vi "Template Retrieve Record.vi"(8 "error in (no error)":errorcluster, 11 "Statement Refnum":T1) -> (0 "error out":errorcluster, 2 "Template Record":T2, 3 "Statement Refnum":T1)   [LabVIEW 2011]
uses:
  Template Record.ctl
  Summitek EXT/ODBC/SQL Controls/Statement Refnum.ctl
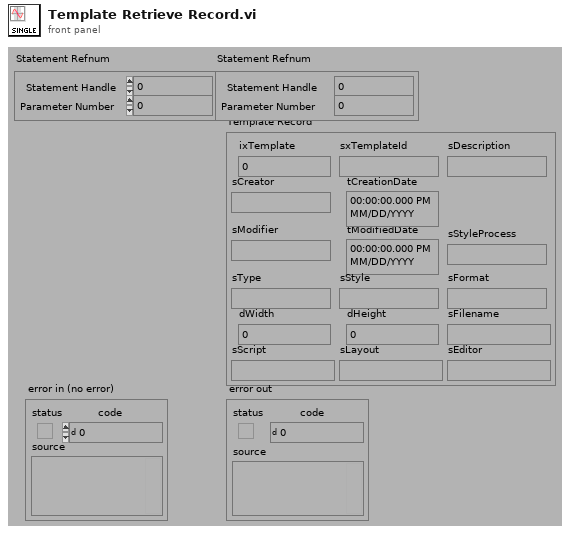
[diagram p1: front panel]
types:
  T1 = typedef "Statement Refnum.ctl" = cluster{"Statement Handle":i32, "Parameter Number":u16}
  T2 = typedef "Template Record.ctl" = cluster{"ixTemplate":i32, "sxTemplateId":string, "sDescription":string, "sCreator":string, "tCreationDate":timestamp, "sModifier":string, "tModifiedDate":timestamp, "sType":string, "sStyle":string, "sFormat":string, "dWidth":dbl, "dHeight":dbl, "sFilename":string, "sScript":string, "sLayout":string, "sEditor":string, "sStyleProcess":string}
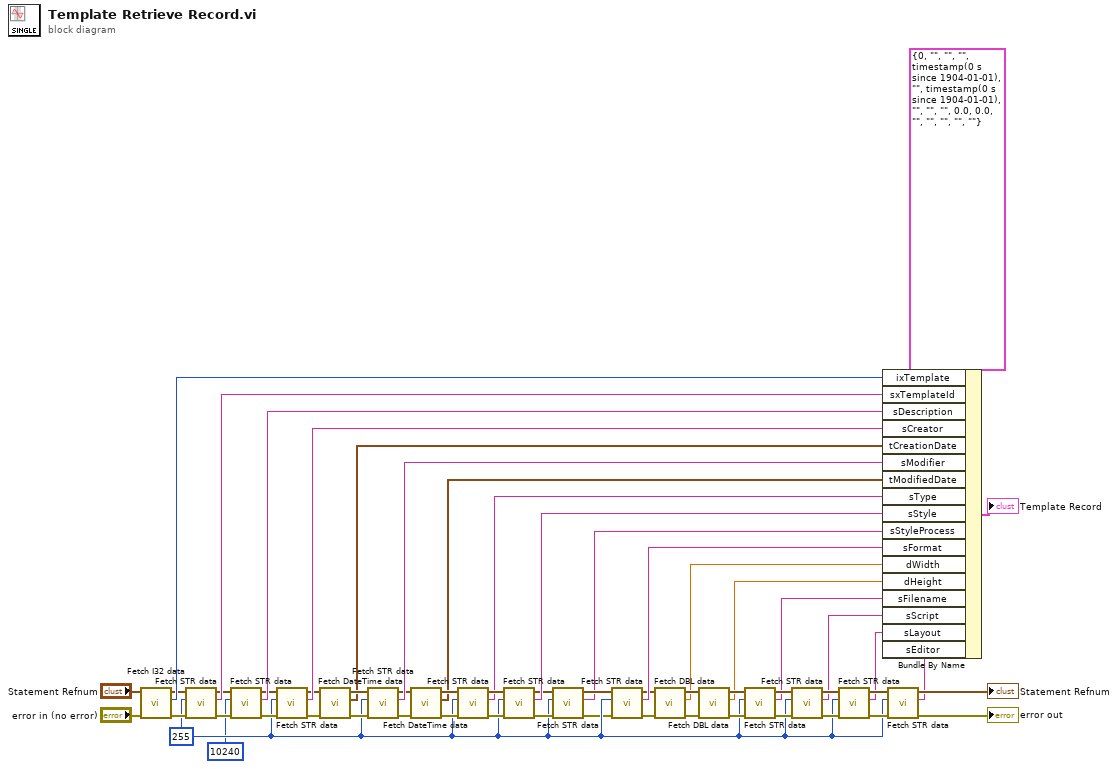
[diagram p0: block diagram]
diagram:
  w5 = 255 ("Buffer Size")
  n1 = call "Fetch I32 data.vi"("error in (no error)"="error in (no error)", "Statement Refnum"="Statement Refnum") -> ("error out"=w35:errorcluster, "Data"=w37:i32, "Statement Refnum"=w36:T1)  [unwired: 3 out]
  n2 = call "Fetch STR data.vi"("error in (no error)"=w35, "Buffer Size"=w5, "Statement Refnum"=w36) -> ("error out"=w33:errorcluster, "Data"=w34:string, "Statement Refnum"=w32:T1)  [unwired: 2 out]
  n3 = call "Fetch STR data.vi"("error in (no error)"=w33, "Buffer Size"=10240, "Statement Refnum"=w32) -> ("error out"=w30:errorcluster, "Data"=w31:string, "Statement Refnum"=w29:T1)  [unwired: 2 out]
  n4 = call "Fetch STR data.vi"("error in (no error)"=w30, "Buffer Size"=w5, "Statement Refnum"=w29) -> ("error out"=w26:errorcluster, "Data"=w28:string, "Statement Refnum"=w27:T1)  [unwired: 2 out]
  n5 = call "Fetch DateTime data.vi"("error in (no error)"=w26, "Statement Refnum"=w27) -> ("error out"=w51:errorcluster, "Data"=w25:timestamp, "Statement Refnum"=w50:T1)  [unwired: 3 out]
  n6 = call "Fetch STR data.vi"("error in (no error)"=w51, "Buffer Size"=w5, "Statement Refnum"=w50) -> ("error out"=w23:errorcluster, "Data"=w24:string, "Statement Refnum"=w22:T1)  [unwired: 2 out]
  n7 = call "Fetch DateTime data.vi"("error in (no error)"=w23, "Statement Refnum"=w22) -> ("error out"=w20:errorcluster, "Data"=w19:timestamp, "Statement Refnum"=w21:T1)  [unwired: 3 out]
  n8 = call "Fetch STR data.vi"("error in (no error)"=w20, "Buffer Size"=w5, "Statement Refnum"=w21) -> ("error out"=w54:errorcluster, "Data"=w16:string, "Statement Refnum"=w53:T1)  [unwired: 2 out]
  n9 = call "Fetch STR data.vi"("error in (no error)"=w54, "Buffer Size"=w5, "Statement Refnum"=w53) -> ("error out"=w6:errorcluster, "Data"=w18:string, "Statement Refnum"=w7:T1)  [unwired: 2 out]
  n10 = call "Fetch STR data.vi"("error in (no error)"=w6, "Buffer Size"=w5, "Statement Refnum"=w7) -> ("error out"=w3:errorcluster, "Data"=w2:string, "Statement Refnum"=w4:T1)  [unwired: 2 out]
  n11 = call "Fetch STR data.vi"("error in (no error)"=w3, "Buffer Size"=w5, "Statement Refnum"=w4) -> ("error out"=w14:errorcluster, "Data"=w17:string, "Statement Refnum"=w15:T1)  [unwired: 2 out]
  n12 = call "Fetch DBL data.vi"("error in (no error)"=w14, "Statement Refnum"=w15) -> ("error out"=w41:errorcluster, "Data"=w13:dbl, "Statement Refnum"=w40:T1)  [unwired: 3 out]
  n13 = call "Fetch DBL data.vi"("error in (no error)"=w41, "Statement Refnum"=w40) -> ("error out"=w38:errorcluster, "Data"=w12:dbl, "Statement Refnum"=w39:T1)  [unwired: 3 out]
  n14 = call "Fetch STR data.vi"("error in (no error)"=w38, "Buffer Size"=w5, "Statement Refnum"=w39) -> ("error out"=w45:errorcluster, "Data"=w11:string, "Statement Refnum"=w49:T1)  [unwired: 2 out]
  n15 = call "Fetch STR data.vi"("error in (no error)"=w45, "Buffer Size"=w5, "Statement Refnum"=w49) -> ("error out"=w44:errorcluster, "Data"=w10:string, "Statement Refnum"=w48:T1)  [unwired: 2 out]
  n16 = call "Fetch STR data.vi"("error in (no error)"=w44, "Buffer Size"=w5, "Statement Refnum"=w48) -> ("error out"=w43:errorcluster, "Data"=w9:string, "Statement Refnum"=w47:T1)  [unwired: 2 out]
  n17 = call "Fetch STR data.vi"("error in (no error)"=w43, "Buffer Size"=w5, "Statement Refnum"=w47) -> ("error out"=→"error out":errorcluster, "Data"=w8:string, "Statement Refnum"=→"Statement Refnum":T1)  [unwired: 2 out]
  n18 = Bundle By Name(cluster=T2 {"ixTemplate"=0, "sxTemplateId"="", "sDescription"="", "sCreator"="", "tCreationDate"=timestamp(0 s since 1904-01-01), "sModifier"="", "tModifiedDate"=timestamp(0 s since 1904-01-01), "sType"="", "sStyle"="", "sFormat"="", "dWidth"=0.0, "dHeight"=0.0, "sFilename"="", "sScript"="", "sLayout"="", "sEditor"="", "sStyleProcess"=""} ("Test Information"), "ixTemplate"=w37, "sxTemplateId"=w34, "sDescription"=w31, "sCreator"=w28, "tCreationDate"=w25, "sModifier"=w24, "tModifiedDate"=w19, "sType"=w16, "sStyle"=w18, "sStyleProcess"=w2, "sFormat"=w17, "dWidth"=w13, "dHeight"=w12, "sFilename"=w11, "sScript"=w10, "sLayout"=w9, "sEditor"=w8) -> (→"Template Record":T2)
